vi "Up Down Counter with Limits.vi"() -> ()   [LabVIEW 2016]
panel:
  out "x 2":dbl
  out "x":dbl
  in  "Boolean":bool
  in  "stop":bool
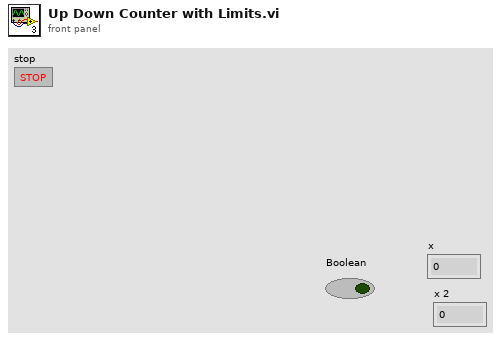
[diagram p1: front panel]
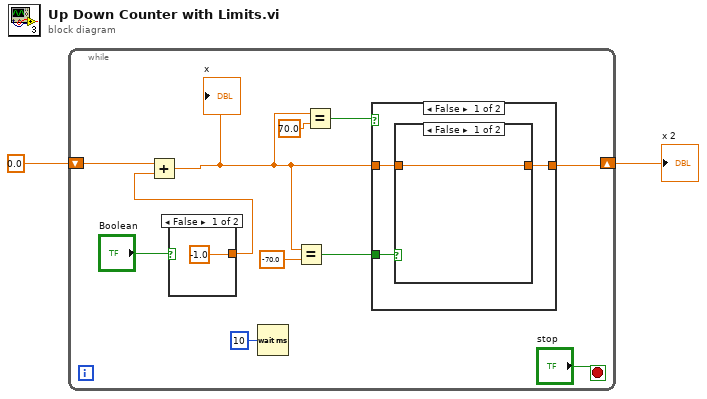
[diagram p0: block diagram]
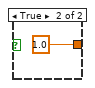
[diagram p2: hidden frame]
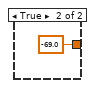
[diagram p3: hidden frame]
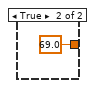
[diagram p4: hidden frame]
diagram:
  n1 = while {
    shift-right: [w9] -> w1
    shift-left: 0.0 ("x") -> [w13]
    stop <- "stop" stop-if-true
    n2 = case shown="False" "Boolean" {
      tunnel: [-1.0 1.0] -> w5
      frame False {
      }
      frame True {
      }
    }
    n3 = Add(x=w13, y=w5) -> (x+y=w4:dbl)
    "x" <- w4
    n4 = Wait (ms)(milliseconds to wait=u32 10) -> ()  [unwired: 1 out]
    n5 = Equal?(x=w4, y=-70.0) -> (x = y?=w3:bool)
    n6 = Equal?(x=w4, y=70.0) -> (x = y?=w10:bool)
    n7 = case shown="False" w10 {
      tunnel: w4 -> [w17 _]
      tunnel: [w16 69.0] -> w9
      tunnel: w3 -> [w18 _]
      frame False {
        n8 = case shown="False" w18 {
          tunnel: w17 -> [w19 _]
          tunnel: [w19 -69.0] -> w16
          frame False {
          }
          frame True {
          }
        }
      }
      frame True {
      }
    }
  }
  "x 2" <- w1
